vi "Preview.vi"(8 "error in (no error)":errorcluster, 10 "Append option":T1, 11 "Scheduler in":refnum<class "Scheduler.lvclass">) -> (0 "error out":errorcluster, 3 "Scheduler out":refnum<class "Scheduler.lvclass">)   [LabVIEW 2020, in "Scheduler.lvlib" / "Scheduler.lvclass"]
uses:
  Scheduler.lvclass
  C:/LabVIEW Code/CIRCUS/TALOS/TALOS_PPL.lvlibp/Father of all uServices/Father of all uServices/Father of all uServices.lvclass
  Run Utilities/Schedule/Array of Runs - GUI.ctl
  Run Utilities/Cell/Cell - GUI.ctl
  Run Utilities/Run Instance/Run Instance - GUI.ctl
  Run Utilities/TypeDefs/Synchronize FPGA Cluster.ctl
  Append Options.ctl
  Scheduler.lvclass/Scheduler.ctl
  Scheduler Consumer Case Selector.ctl
  TALOS/TALOS_PPL.lvlibp/Guardian/Guardian/Requests.ctl
  TALOS/TALOS_PPL.lvlibp/Father of all uServices/Father of all uServices/Children Methods/Get GUI Item Value - Variant.vi
  TALOS/TALOS_PPL.lvlibp/Support VIs/Global Constants.vi
  Run Utilities/Sequence of SBlocks/Sequence of SBlocks.lvclass
  Run Utilities/Schedule/Schedule.lvclass
  Run Utilities/Run Utilities.lvlib
  Scheduling_gif.vi
  Abort_gif.vi
  TALOS/TALOS_PPL.lvlibp/Father of all uServices/Father of all uServices/Father of all uServices.lvclass
  TALOS/TALOS_PPL.lvlibp
  TALOS/TALOS_PPL.lvlibp/Guardian/Guardian/Guardian.lvclass
  C:/LabVIEW Code/CIRCUS/TALOS/TALOS_PPL.lvlibp/Ancestor/Ancestor/Ancestor.lvclass
  C:/LabVIEW Code/CIRCUS/TALOS/Actor Framework.lvlibp/1abvi3w/vi.lib/ActorFramework/Actor/Actor.lvclass
  C:/LabVIEW Code/CIRCUS/CIRCUS uServices et al/Scheduler/Scheduler.lvclass
  Run Utilities/Run Instance/Run Instance.lvclass
  Run Utilities/Cell/Schedule Cell.lvclass
panel:
  out "Sync. Mask":T2[](array[typedef])
  in  "ACCEPT":bool
  in  "CANCEL":bool
  out "Prepared Schedules":cluster{"Continuous":bool, "Array of Runs":T3}[](array[cluster]) {"Array of Runs"."Number of cycles" min=1}
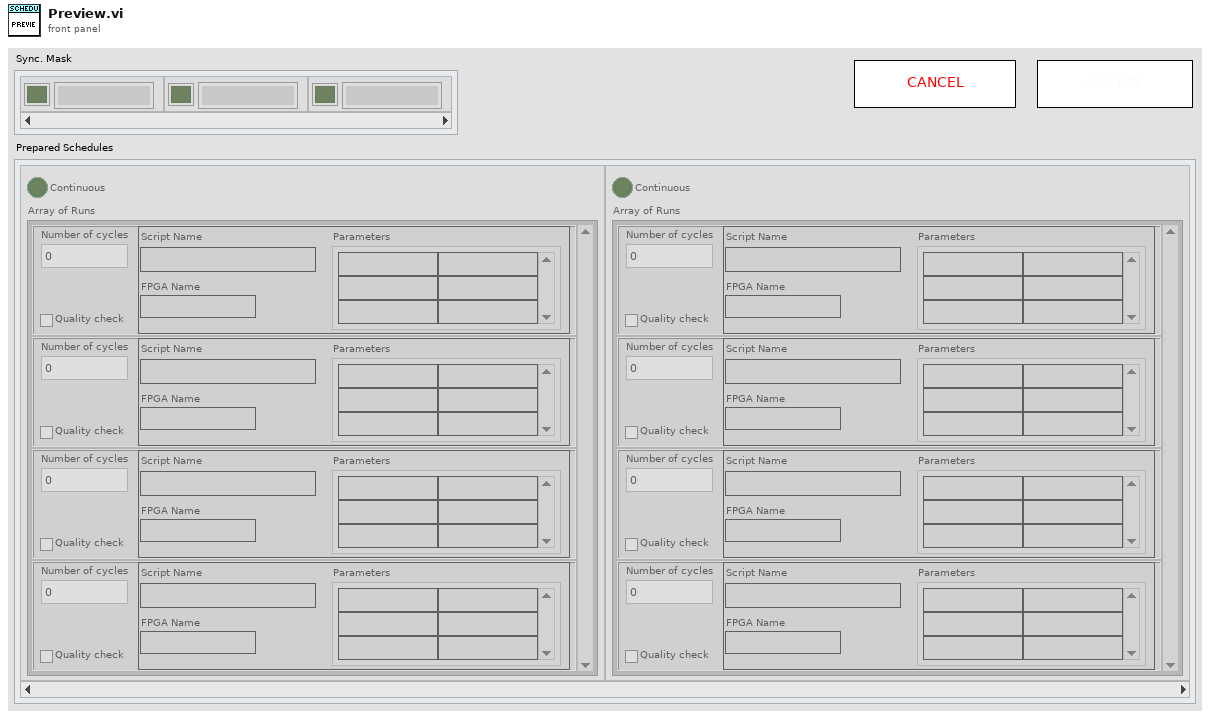
[diagram p1: front panel]
types:
  T1 = typedef "Scheduler.lvlib/Scheduler.lvclass/Append Options.ctl" = enum16{"New session", "Append to bottom", "Append to top"}
  T2 = typedef "Run Utilities.lvlib/Synchronize FPGA Cluster.ctl" = cluster{"Status":bool, "FPGA Name":string}
  T3 = typedef "Run Utilities.lvlib/Schedule.lvclass/Array of Runs - GUI.ctl" = T4[]
  T4 = typedef "Run Utilities.lvlib/Schedule Cell.lvclass/Cell - GUI.ctl" = cluster{"Background Color":u32, "Number of cycles":u32, "Single RUN":T5, "Quality check":bool, "Cell Type":string}
  T5 = typedef "Run Utilities.lvlib/Run Instance.lvclass/Run Instance - GUI.ctl" = cluster{"Script Name":string, "Parameters":string[][], "FPGA Name":string}
  T6 = enum8{"Enabled", "Disabled", "Disabled and Grayed Out"}
  T7 = typedef "TALOS_PPL.lvlibp/Guardian.lvlib/Guardian.lvclass/Requests.ctl" = enum16{"Ready to Launch", "Start RUN", "Stop RUN", "Update DAQ Params", "Update Error Listbox", "Update Run Status", "Update Kasli Log", "Run Stopped with Errors", "Switch uS View"}
  T8 = typedef "Scheduler.lvlib/Scheduler.lvclass/Scheduler Consumer Case Selector.ctl" = enum16{"Add SBlock", "Update GUI", "Move SBlock", "Select SBlock", "Update Cont.", "Load", "Save", "Reset", "Send to Tamer", "Edit SBlock", "Duplicate SBlock", "Delete SBlock", "Update SBlock", "Init", "Split/Combine Schedules", "Reschedule", "Load Parameters"}
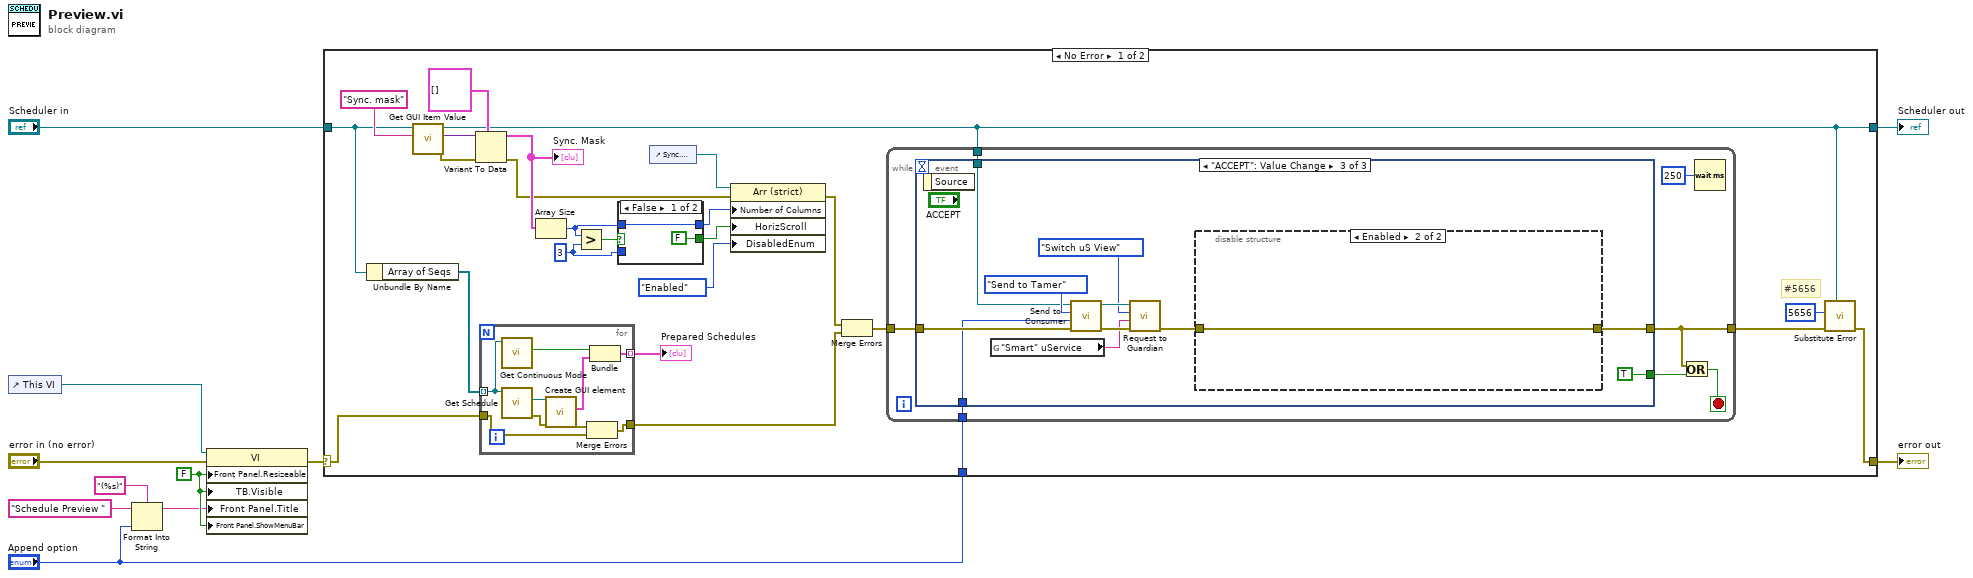
[diagram p0: block diagram]
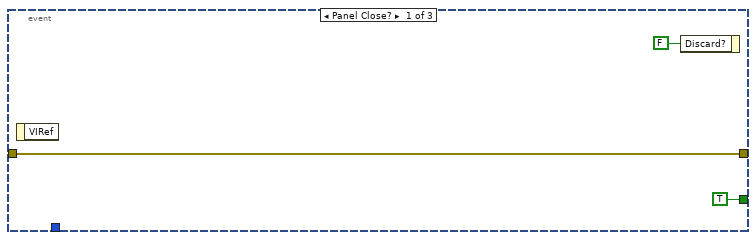
[diagram p2: hidden frame]
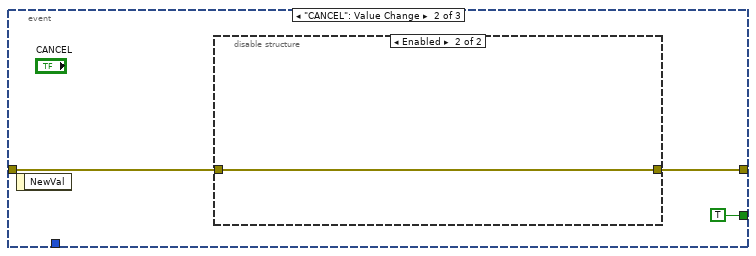
[diagram p3: hidden frame]
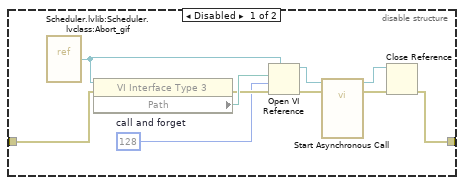
[diagram p4: hidden frame]
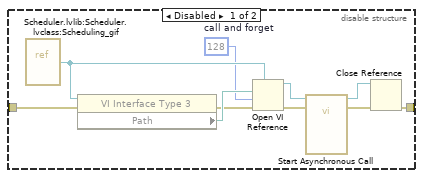
[diagram p5: hidden frame]
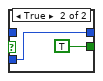
[diagram p6: hidden frame]
diagram:
  w7 = FALSE ("Front Panel Window:Resizable")
  n1 = control-ref of="This VI"() -> (w8:refnum<vi>)
  n2 = Format Into String(format string="(%s)", initial string="Schedule Preview " ("Front Panel Window:Title"), "Append option") -> (resulting string=w2:string)  [unwired: 1 in, 1 out]
  n3 = property class="VI"(reference=w8, error in="error in (no error)", "Front Panel.Resizeable"=w7, "TB.Visible"=w7, "Front Panel.Title"=w2, "Front Panel.ShowMenuBar"=w7) -> (error out=w5:errorcluster)  [unwired: 1 out]
  n4 = case shown="No Error" w5 {
    selector: w5 -> [w35 w97]
    tunnel: [w16 w97] -> w11
    tunnel: [w15 w96] -> w9
    tunnel: "Scheduler in" -> [w13 w96]
    tunnel: "Append option" -> [w12 _]
    frame No Error {
      w25 = 3 ("y")
      # "#5656"
      n5 = Unbundle By Name(w13) -> ("Array of Seqs"=w36:refnum<class "Sequence of SBlocks.lvclass">[])
      n6 = call-poly "Get GUI Item Value.vi"("FP Item Name"="Sync. mask", "uService Template in"=w13) -> ("error out"=w31:errorcluster, "Value"=w33:variant, "uService Template out"=w15:refnum<class "Scheduler.lvclass">)  [unwired: 7 in]
      n7 = Variant To Data(error in=w31, type=T2[] [], Variant=w33) -> (data=w23:T2[], error out=w21:errorcluster)
      "Sync. Mask" <- w23
      n8 = for {
        tunnel: w36 -> [w91] mode=indexing
        tunnel: w35 -> [w84]
        tunnel: [w87] -> w30 mode=indexing
        tunnel: [w86] -> w19
        n9 = call-dynamic "Get Continuous Mode.vi"("Sequence of SBlocks in"=w91) -> ("Continuous"=w90:bool)  [unwired: 8 in, 2 out]
        n10 = call-dynamic "Get Schedule.vi"("Sequence of SBlocks in"=w91) -> ("error out"=w88:errorcluster, "Schedule"=w83:refnum<class "Schedule.lvclass">)  [unwired: 8 in, 1 out]
        n11 = call-dynamic "Create GUI element.vi"("error in (no error)"=w88, "Schedule in"=w83) -> ("error out"=w85:errorcluster, "Array of Runs"=w89:T3)  [unwired: 7 in, 1 out]
        n12 = Merge Errors(w85, w84) -> (w86:errorcluster)
        n13 = Bundle("Continuous"=w90, "Array of Runs"=w89) -> (w87:cluster{"Continuous":bool, "Array of Runs":T3})  [unwired: 1 in]
      }
      "Prepared Schedules" <- w30
      n14 = Array Size(array=w23) -> (size(s)=w29:i32)
      n15 = Greater?(x=w29, y=w25) -> (0:w26:bool)
      n16 = case shown="False" w26 {
        tunnel: [w92 w94] -> w27
        tunnel: [FALSE TRUE] -> w28
        tunnel: w29 -> [w92 _]
        tunnel: w25 -> [_ w94]
        frame False {
        }
        frame True {
        }
      }
      n17 = control-ref of="Sync. Mask"() -> (w22:refnum<vi>)
      n18 = property class="Arr (strict)"(reference=w22, error in=w21, "Number of Columns"=w27, "HorizScroll"=w28, "DisabledEnum"=T6."Enabled" ("Disabled")) -> (error out=w20:errorcluster)  [unwired: 1 out]
      n19 = Merge Errors(w20, w19) -> (w18:errorcluster)
      n20 = while {
        tunnel: w18 -> [w42]
        tunnel: [w39] -> w17
        tunnel: w15 -> [w38]
        tunnel: w12 -> [w37]
        stop <- w41 stop-if-true
        n21 = event shown="[2] \"ACCEPT\": Value Change" {
          selector: _ -> [_ _ _]
          dyn-events: _ -> [_ _ _]
          timeout: _ -> [_ _ _]
          tunnel: w42 -> [w45 w47 w70]
          tunnel: [w45 w48 w68] -> w39
          tunnel: [TRUE TRUE TRUE] -> w40
          tunnel: w38 -> [_ _ w62]
          tunnel: w37 -> [_ _ w61]
          event Panel Close? {
            n22 = event-data() -> ()  [unwired: 1 in, 1 out]
            n23 = event-data("Discard?"=FALSE) -> ()  [unwired: 1 in, 1 out]
          }
          event "CANCEL": Value Change {
            n24 = event-data() -> ()  [unwired: 1 in, 1 out]
            n25 = disable-structure shown="Enabled" {
              disable-tunnel: [w51 w60] -> w48
              disable-tunnel: w47 -> [w50 w60]
              frame Disabled {
                w52 = 128  # call and forget
                n26 = vi-ref "Scheduler.lvlib:Scheduler.lvclass:Abort_gif.vi"() -> (w58:refnum<vi>)
                n27 = property class="VI Interface Type 3"(reference=w58, error in=w50) -> (error out=w53:errorcluster, "Path"=w54:path)  [unwired: 1 out]
                n28 = Open VI Reference(type specifier VI Refnum (for type only)=w58, vi path=w54, options=w52, error in (no error)=w53) -> (vi reference=w56:refnum<vi>, error out=w59:errorcluster)  [unwired: 2 in]
                n29 = call-by-ref "Start Asynchronous Call"(reference=w56, error in=w59) -> (reference out=w55:refnum<vi>, error out=w57:errorcluster)  [unwired: 12 in]
                n30 = Close Reference(reference=w55, error in (no error)=w57) -> (error out=w51:errorcluster)
              }
              frame Enabled {
              }
            }
          }
          event "ACCEPT": Value Change {
            n31 = event-data() -> ()  [unwired: 1 in, 1 out]
            n32 = global read "Global Constants.vi" "\"Smart\" uService"() -> (w63:string)
            n33 = call "Send to Consumer.vi"("error in (no error)"=w70, "Data"=w61, "Case ID"=Scheduler_Consumer_Case_Selector."Send to Tamer" ("Shifter Panel Consumer Case Selector"), "uService Template in"=w62) -> ("error out"=w67:errorcluster, "uService Template out"=w65:refnum<class "Scheduler.lvclass">)  [unwired: 6 in]
            n34 = call "Request to Guardian.vi"("error in (no error)"=w67, "Data"=w63, "Requests"=Requests."Switch uS View", "Father of all uServices in"=w65) -> ("error out"=w66:errorcluster)  [unwired: 6 in, 1 out]
            n35 = disable-structure shown="Enabled" {
              disable-tunnel: [w73 w82] -> w68
              disable-tunnel: w66 -> [w72 w82]
              frame Disabled {
                w74 = 128  # call and forget
                n36 = vi-ref "Scheduler.lvlib:Scheduler.lvclass:Scheduling_gif.vi"() -> (w80:refnum<vi>)
                n37 = property class="VI Interface Type 3"(reference=w80, error in=w72) -> (error out=w75:errorcluster, "Path"=w76:path)  [unwired: 1 out]
                n38 = Open VI Reference(type specifier VI Refnum (for type only)=w80, vi path=w76, options=w74, error in (no error)=w75) -> (vi reference=w78:refnum<vi>, error out=w81:errorcluster)  [unwired: 2 in]
                n39 = call-by-ref "Start Asynchronous Call"(reference=w78, error in=w81) -> (reference out=w77:refnum<vi>, error out=w79:errorcluster)  [unwired: 12 in]
                n40 = Close Reference(reference=w77, error in (no error)=w79) -> (error out=w73:errorcluster)
              }
              frame Enabled {
              }
            }
          }
        }
        n41 = Or(x=w39, y=w40) -> (x .or. y?=w41:bool)
        n42 = Wait (ms)(milliseconds to wait=u32 250) -> ()  [unwired: 1 out]
      }
      n43 = call "Substitute Error.vi"("LabVIEW Object"=w15, "error in (no error)"=w17, "Error Code"=5656) -> ("error out"=w16:errorcluster)  [unwired: 8 in]
    }
    frame Error {
    }
  }
  "error out" <- w11
  "Scheduler out" <- w9
